vi "Pad Advanced Settings.vi"(8 "Error In":errorcluster) -> (0 "Error Out":errorcluster, 2 "Ok?":bool, 3 "Path to Calibration File":path)   [LabVIEW 2014]
doc: "This VI provides advanced settings like calibration and choosing buttons for game controllers"
uses:
  Controls/Controllers Clusters/Game Pad Buttons Cluster.ctl
  Controls/Controllers Clusters/Pad Advanced Settings States.ctl
  Controls/Controllers Clusters/Game Pad Calibration Cluster.ctl
  Controls/Configuration Files.ctl
  <vilib>/Utility/xml.llb/Read From XML File(string).vi
  <vilib>/Utility/inputDevices.llb/closeJoystick.vi
  <vilib>/Utility/inputDevices.llb/joystickAcquire.vi
panel:
  in  "Load Button":bool
  out "V Axis":i32(slide) scale=-32768.0..32767.0
  out "U Axis":i32(slide) scale=-32768.0..32767.0
  in  "Calibration Button":bool
  out "Buttons":T1
  out "Z Axis Rotation":i32(slide) scale=-32768.0..32767.0
  out "Y Axis Rotation":i32(slide) scale=-32768.0..32767.0
  out "Y Axis":i32(slide) scale=-32768.0..32767.0
  out "X Axis":i32(slide) scale=-32768.0..32767.0
  out "Z Axis":i32(slide) scale=-32768.0..32767.0
  out "X Axis Rotation":i32(slide) scale=-32768.0..32767.0
  in  "Connect Button":bool
  in  "Cancel Button":bool
  in  "OK Button":bool
  # "Game Controllers Advanced Settings"
  # "OK will be available if Path to Calibration File will be correct"
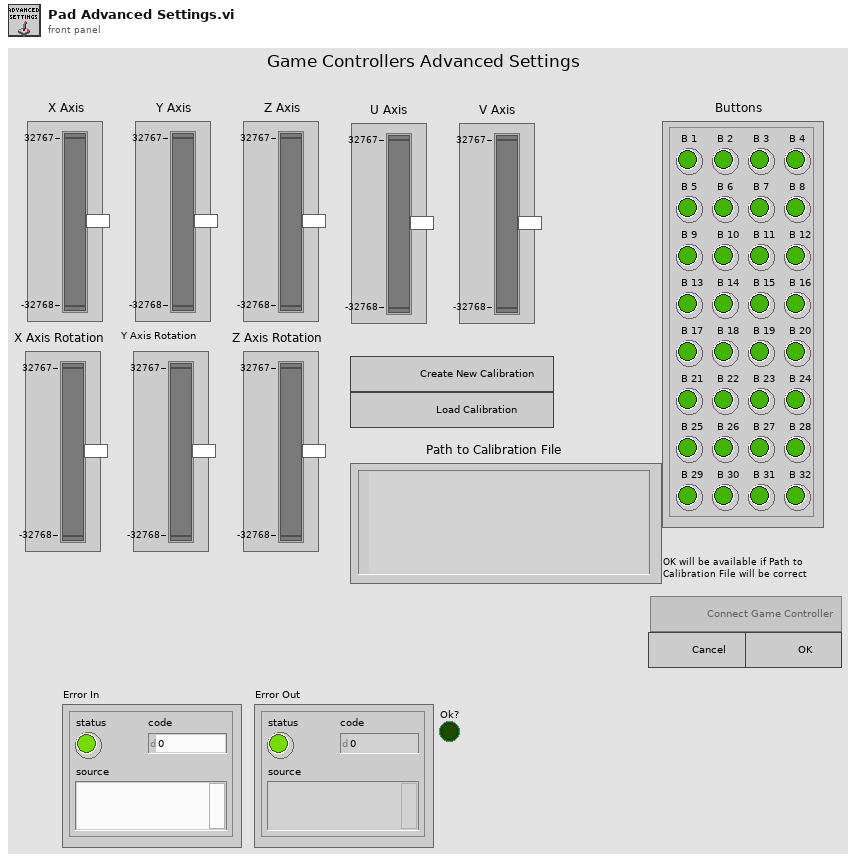
[diagram p1: front panel]
types:
  T1 = typedef "Game Pad Buttons Cluster.ctl" = cluster{"B 1":bool, "B 2":bool, "B 3":bool, "B 4":bool, "B 5":bool, "B 6":bool, "B 7":bool, "B 8":bool, "B 9":bool, "B 10":bool, "B 11":bool, "B 12":bool, "B 13":bool, "B 14":bool, "B 15":bool, "B 16":bool, "B 17":bool, "B 18":bool, "B 19":bool, "B 20":bool, "B 21":bool, "B 22":bool, "B 23":bool, "B 24":bool, "B 25":bool, "B 26":bool, "B 27":bool, "B 28":bool, "B 29":bool, "B 30":bool, "B 31":bool, "B 32":bool}
  T2 = typedef "Pad Advanced Settings States.ctl" = enum16{"Init", "Wait for Event", "Ok", "Cancel"}
  T3 = enum8{"Enabled", "Disabled", "Disabled and Grayed Out"}
  T4 = typedef "Configuration Files.ctl" = string
  T5 = cluster{"X axis":i32, "Y axis":i32, "Z axis":i32, "X axis rotation":i32, "Y axis rotation":i32, "Z axis rotation":i32, "U axis":i32, "V axis":i32}
  T6 = cluster{"button 1":bool, "button 2":bool, "button 3":bool, "button 4":bool, "button 5":bool, "button 6":bool, "button 7":bool, "button 8":bool, "button 9":bool, "button 10":bool, "button 11":bool, "button 12":bool, "button 13":bool, "button 14":bool, "button 15":bool, "button 16":bool, "button 17":bool, "button 18":bool, "button 19":bool, "button 20":bool, "button 21":bool, "button 22":bool, "button 23":bool, "button 24":bool, "button 25":bool, "button 26":bool, "button 27":bool, "button 28":bool, "button 29":bool, "button 30":bool, "button 31":bool, "button 32":bool}
  T7 = typedef "Game Pad Calibration Cluster.ctl" = cluster{"Safety Button Number":u8, "Speed Axis Number":u8, "Speed Axis Max":i32, "Speed Axis Zero":i32, "Back Speed Axis Number":u8, "Back Speed Axis Max":i32, "Back Speed Axis Zero":i32, "Steering Axis Number":u8, "Steering Axis Max":i32, "Steering Axis Zero":i32}
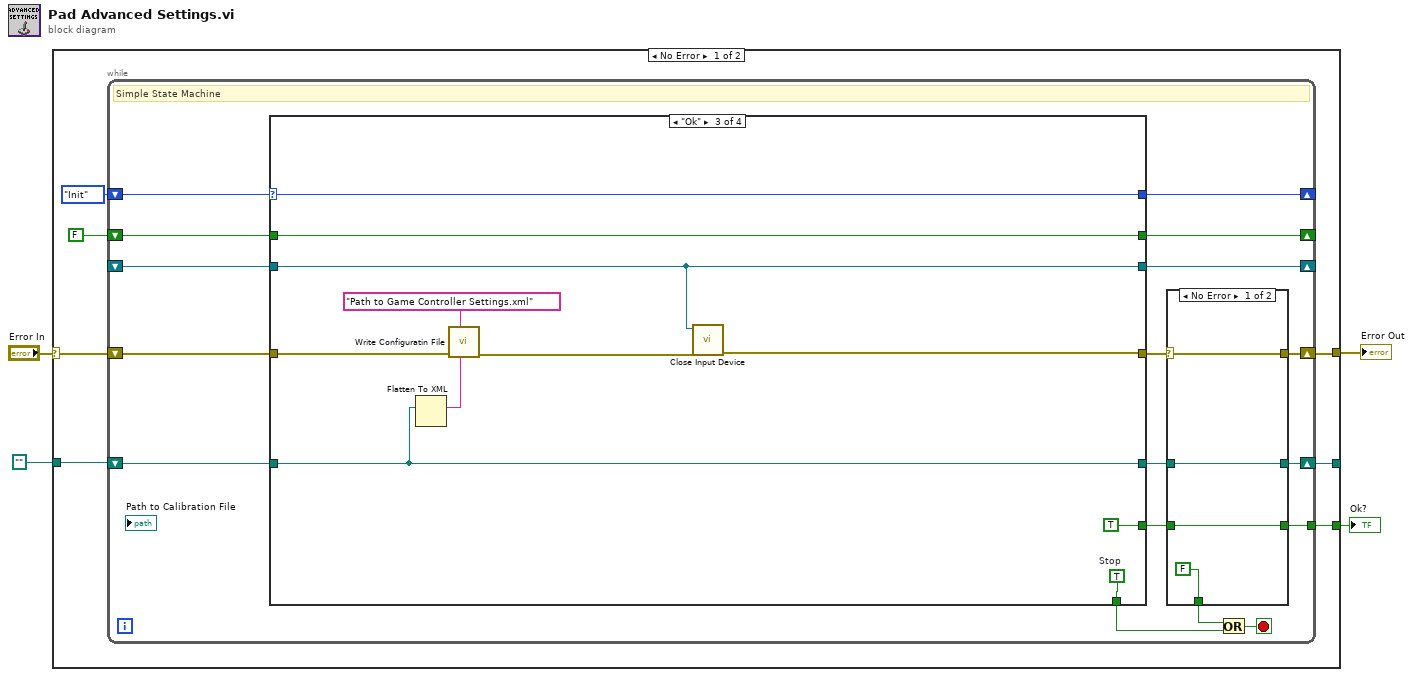
[diagram p0: block diagram]
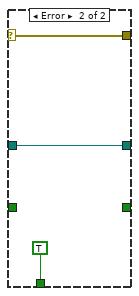
[diagram p2: hidden frame]
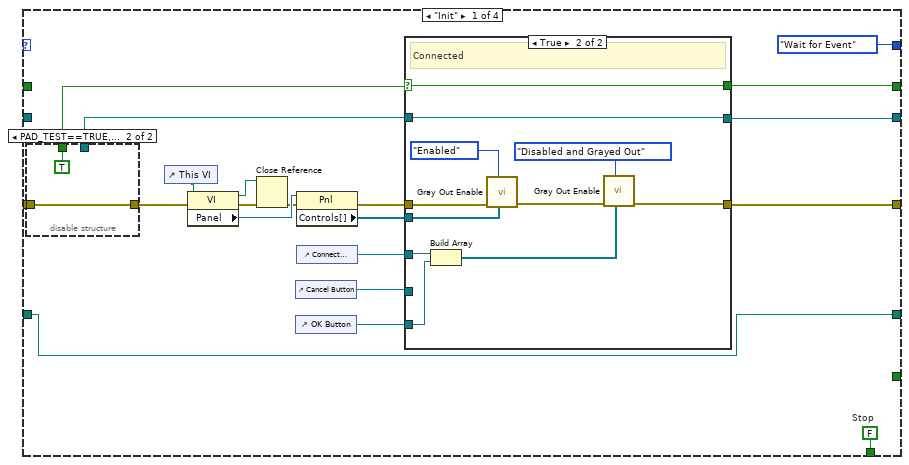
[diagram p3: hidden frame]
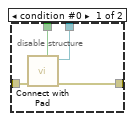
[diagram p4: hidden frame]
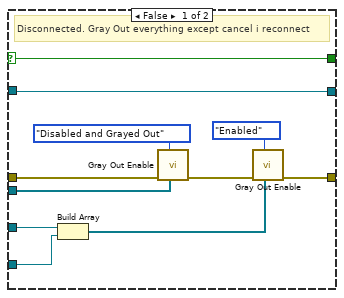
[diagram p5: hidden frame]
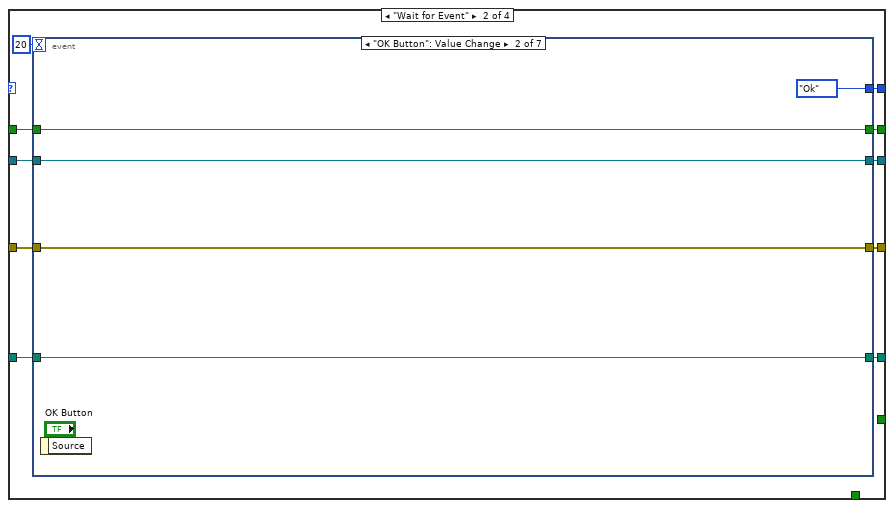
[diagram p6: hidden frame]
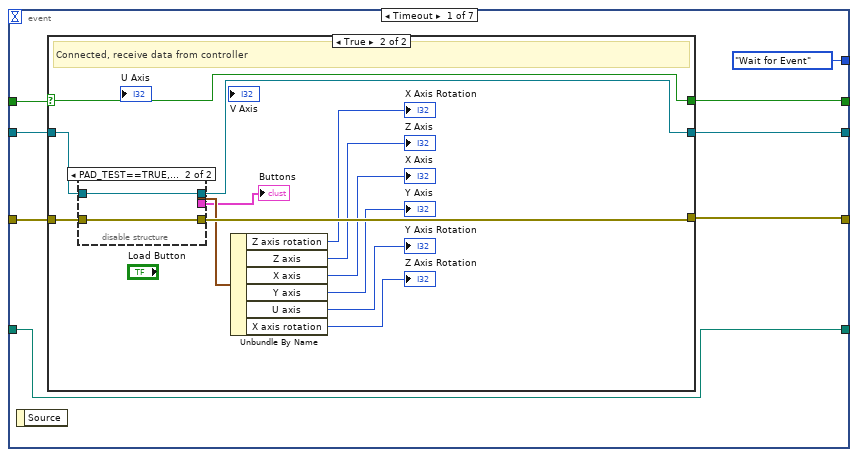
[diagram p7: hidden frame]
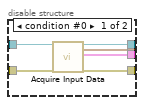
[diagram p9: hidden frame]
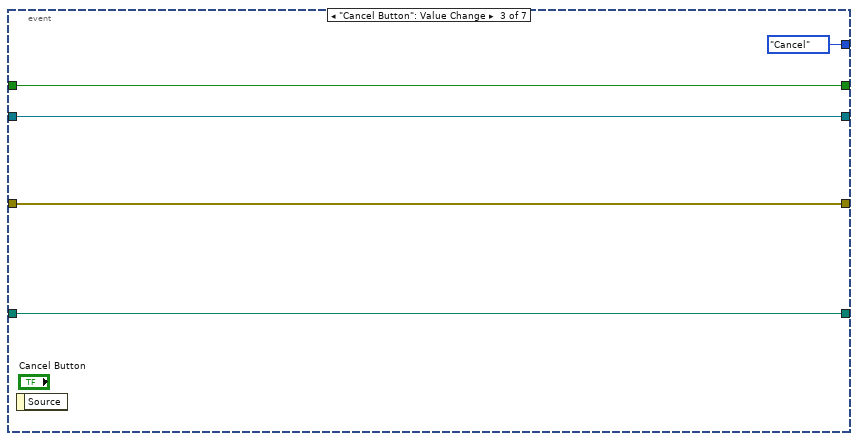
[diagram p10: hidden frame]
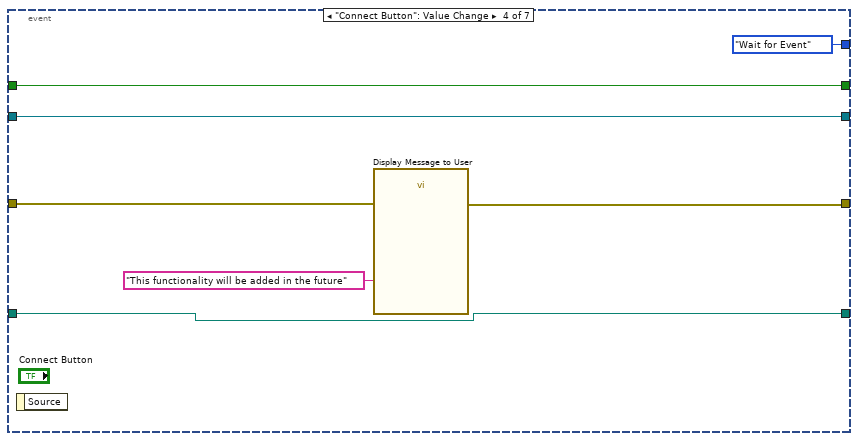
[diagram p11: hidden frame]
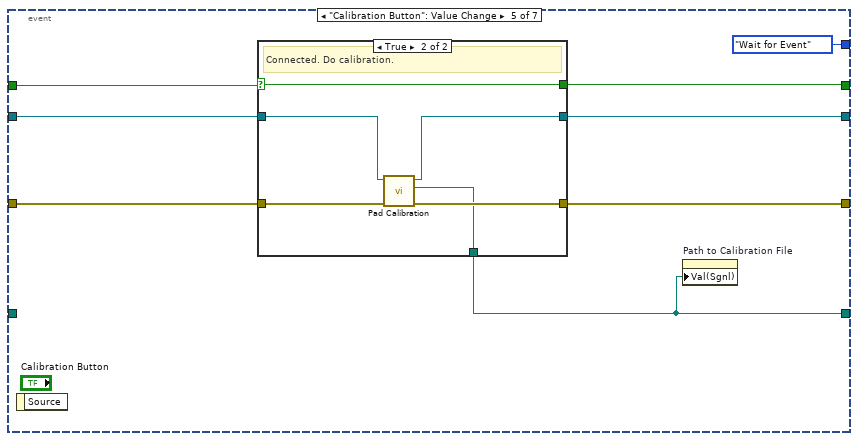
[diagram p12: hidden frame]
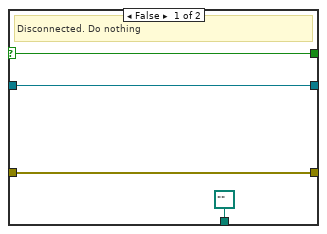
[diagram p13: hidden frame]
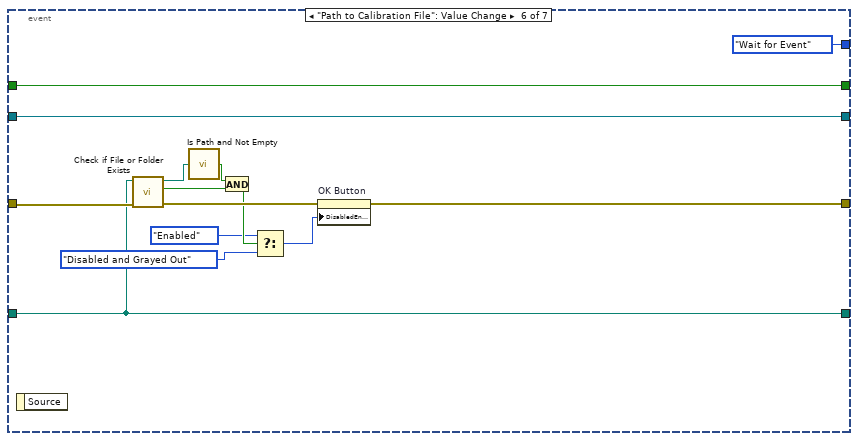
[diagram p14: hidden frame]
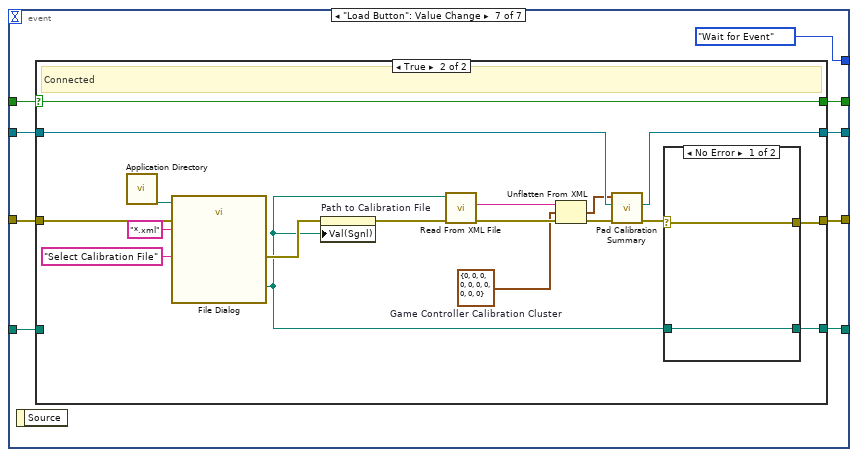
[diagram p15: hidden frame]
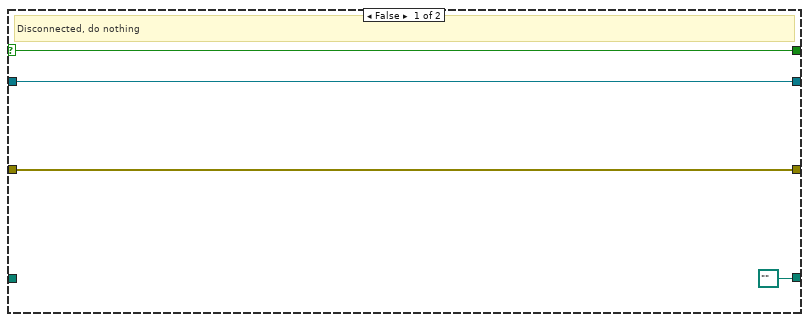
[diagram p16: hidden frame]
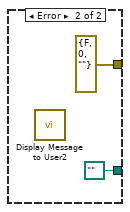
[diagram p17: hidden frame]
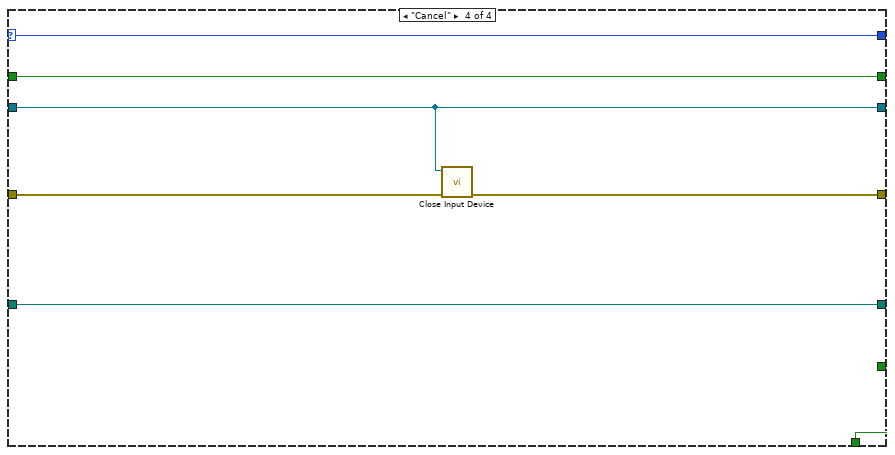
[diagram p18: hidden frame]
diagram:
  n1 = case shown="No Error" "Error In" {
    selector: "Error In" -> [w10 w229]
    tunnel: [w9 w229] -> w3
    tunnel: [w7 w228] -> _
    tunnel: path "" -> [w6 w228]
    tunnel: [w5 _] -> w1
    frame No Error {
      n2 = while {
        shift-right: [w25] -> w9
        shift-left: w10 -> [w14]
        shift-right: [w27] -> _
        shift-left: Pad_Advanced_Settings_States."Init" -> [w28]
        shift-right: [w20] -> _
        shift-left: FALSE -> [w21]
        shift-right: [w18] -> _
        shift-left: _ -> [w19]
        shift-right: [w16] -> w7
        shift-left: w6 -> [w15]
        tunnel: [w12] -> w5
        stop <- w24 stop-if-true
        # "Simple State Machine"
        n3 = case shown="\"Ok\"" w28 {
          selector: w28 -> [_ _ w220 w226]
          tunnel: w14 -> [w53 w93 w215 w223]
          tunnel: [w40 w92 w217 w224] -> w26
          tunnel: [w55 _ w219 w227] -> w22
          tunnel: [Pad_Advanced_Settings_States."Wait for Event" w91 w220 w226] -> w27
          tunnel: w21 -> [_ w90 w218 w225]
          tunnel: [w38 w89 w218 w225] -> w20
          tunnel: [w39 w87 w216 w222] -> w18
          tunnel: w19 -> [_ w88 w216 w222]
          tunnel: [w36 w85 w212 w221] -> w17
          tunnel: w15 -> [w36 w84 w212 w221]
          tunnel: [_ _ TRUE _] -> w13
          frame "Init" {
            w55 = FALSE  # Stop
            n4 = disable-structure shown="PAD_TEST==TRUE, Default" {
              disable-tunnel: w53 -> [w59 w61]
              disable-tunnel: [w58 TRUE ("Connected?")] -> w43
              disable-tunnel: [w57 _] -> w42
              disable-tunnel: [w56 w61] -> w41
              frame condition #0 {
                n5 = call "Connect with Pad.vi"("error in (no error)"=w59) -> ("error out"=w56:errorcluster, "device ID"=w57:refnum<k1>, "Connected?"=w58:bool)  [unwired: 8 in]
              }
              frame condition #1 (active) {
              }
            }
            n6 = control-ref of="This VI"() -> (w48:refnum<vi>)
            n7 = property class="VI"(reference=w48, error in=w41) -> (reference out=w51:refnum<vi>, error out=w50:errorcluster, "Panel"=w52:refnum<vi>)
            n8 = Close Reference(reference=w51, error in (no error)=w50) -> (error out=w49:errorcluster)
            n9 = control-ref of="Cancel Button"() -> (w44:refnum<vi>)
            n10 = control-ref of="OK Button"() -> (w37:refnum<vi>)
            n11 = property class="Pnl"(reference=w52, error in=w49) -> (error out=w47:errorcluster, "Controls[]"=w46:refnum<vi>[])  [unwired: 1 out]
            n12 = control-ref of="Connect Button"() -> (w45:refnum<vi>)
            n13 = case shown="True" w43 {
              selector: w43 -> [w72 w83]
              tunnel: [w72 w83] -> w38
              tunnel: [w71 w82] -> w39
              tunnel: w42 -> [w71 w82]
              tunnel: w47 -> [w65 w81]
              tunnel: [w68 w74] -> w40
              tunnel: w46 -> [w66 w79]
              tunnel: w44 -> [w64 _]
              tunnel: w45 -> [w63 w77]
              tunnel: w37 -> [_ w73]
              frame False {
                # "Disconnected. Gray Out everything except cancel i reconnect"
                n14 = Build Array(w63, w64) -> (w62:refnum<vi>[])
                n15 = call "Gray Out Enable.vi"("Controls[]"=w66, "Disabled"=T3."Disabled and Grayed Out", "Error In"=w65) -> ("Error Out"=w69:errorcluster)  [unwired: 8 in]
                n16 = call "Gray Out Enable.vi"("Controls[]"=w62, "Disabled"=T3."Enabled", "Error In"=w69) -> ("Error Out"=w68:errorcluster)  [unwired: 8 in]
              }
              frame True {
                # "Connected"
                n17 = Build Array(w77, w73) -> (w76:refnum<vi>[])
                n18 = call "Gray Out Enable.vi"("Controls[]"=w79, "Disabled"=T3."Enabled", "Error In"=w81) -> ("Error Out"=w75:errorcluster)  [unwired: 8 in]
                n19 = call "Gray Out Enable.vi"("Controls[]"=w76, "Disabled"=T3."Disabled and Grayed Out", "Error In"=w75) -> ("Error Out"=w74:errorcluster)  [unwired: 8 in]
              }
            }
          }
          frame "Wait for Event" {
            n20 = event shown="[1] \"OK Button\": Value Change" {
              selector: _ -> [_ _ _ _ _ _ _]
              dyn-events: _ -> [_ _ _ _ _ _ _]
              timeout: 20 -> [_ _ _ _ _ _ _]
              tunnel: w93 -> [w96 w130 w134 w142 w145 w174 w182]
              tunnel: [w95 w130 w134 w141 w144 w165 w183] -> w92
              tunnel: [Pad_Advanced_Settings_States."Wait for Event" Pad_Advanced_Settings_States."Ok" Pad_Advanced_Settings_States."Cancel" Pad_Advanced_Settings_States."Wait for Event" Pad_Advanced_Settings_States."Wait for Event" Pad_Advanced_Settings_States."Wait for Event" Pad_Advanced_Settings_States."Wait for Event"] -> w91
              tunnel: [w99 w128 w133 w140 w147 w162 w178] -> w89
              tunnel: w90 -> [w101 w128 w133 w140 w149 w162 w179]
              tunnel: w88 -> [w98 w127 w132 w139 w148 w163 w181]
              tunnel: [w97 w127 w132 w139 w146 w163 w180] -> w87
              tunnel: [w94 w126 w131 w136 w143 w164 w176] -> w85
              tunnel: w84 -> [w94 w126 w131 w136 _ w164 w175]
              event Timeout {
                n21 = event-data() -> ()  [unwired: 1 in, 1 out]
                n22 = case shown="True" w101 {
                  selector: w101 -> [w104 w111]
                  tunnel: [w104 w111] -> w99
                  tunnel: w98 -> [w103 w115]
                  tunnel: [w103 w110] -> w97
                  tunnel: [w102 w116] -> w95
                  tunnel: w96 -> [w102 w117]
                  frame False {
                    # "Not connected, do nothing"
                  }
                  frame True {
                    # "Connected, receive data from controller"
                    n23 = disable-structure shown="PAD_TEST==TRUE, Default" {
                      disable-tunnel: w117 -> [w123 w124]
                      disable-tunnel: [w122 w124] -> w116
                      disable-tunnel: w115 -> [w121 w125]
                      disable-tunnel: [w120 _] -> w114
                      disable-tunnel: [w119 w125] -> w110
                      disable-tunnel: [w118 _] -> w105
                      frame condition #0 {
                        n24 = call-poly <vilib>:"Acquire Input Data.vi"("device ID"=w121, "error in (no error)"=w123) -> ("device ID"=w119:refnum<k1>, "axis info"=w120:T5, "button info"=w118:T6, "error out"=w122:errorcluster)  [unwired: 13 in, 1 out]
                      }
                      frame condition #1 (active) {
                      }
                    }
                    "Buttons" <- w105
                    n25 = Unbundle By Name(w114) -> ("Z axis rotation"=→"X Axis Rotation":i32, "Z axis"=→"Z Axis":i32, "X axis"=→"X Axis":i32, "Y axis"=→"Y Axis":i32, "U axis"=→"Y Axis Rotation":i32, "X axis rotation"=→"Z Axis Rotation":i32)
                  }
                }
              }
              event "OK Button": Value Change {
                n26 = event-data() -> ()  [unwired: 1 in, 1 out]
              }
              event "Cancel Button": Value Change {
                n27 = event-data() -> ()  [unwired: 1 in, 1 out]
              }
              event "Connect Button": Value Change {
                n28 = event-data() -> ()  [unwired: 1 in, 1 out]
                n29 = call "Display Message to User"("error in (no error)"=w142, "Message"="This functionality will be added in the future") -> ("error out"=w141:errorcluster)  [unwired: 8 in, 1 out]
              }
              event "Calibration Button": Value Change {
                n30 = event-data() -> ()  [unwired: 1 in, 1 out]
                n31 = case shown="True" w149 {
                  selector: w149 -> [w154 w160]
                  tunnel: w148 -> [w153 w156]
                  tunnel: [w154 w160] -> w147
                  tunnel: [w153 w157] -> w146
                  tunnel: w145 -> [w152 w159]
                  tunnel: [w152 w158] -> w144
                  tunnel: [path "" ("Path to config file") w155] -> w143
                  frame False {
                    # "Disconnected. Do nothing"
                  }
                  frame True {
                    # "Connected. Do calibration."
                    n32 = call "Pad Calibration.vi"("Error In"=w159, "device ID"=w156) -> ("Error Out"=w158:errorcluster, "Path to config file"=w155:path, "device ID"=w157:refnum<k1>)  [unwired: 7 in]
                  }
                }
                n33 = property on="Path to Calibration File" class="Path"("Val(Sgnl)"=w143) -> ()  [unwired: 2 in, 2 out]
              }
              event "Path to Calibration File": Value Change {
                n34 = event-data() -> ()  [unwired: 1 in, 1 out]
                n35 = call <vilib>:"Check if File or Folder Exists.vi"("error in (no error)"=w174, "path"=w164) -> ("error out"=w170:errorcluster, "file or folder exists?"=w171:bool, "dup path"=w173:path)  [unwired: 7 in]
                n36 = call <vilib>:"Is Path and Not Empty.vi"("path"=w173) -> ("Is Path and Not Empty?"=w172:bool)  [unwired: 4 in]
                n37 = And(x=w172, y=w171) -> (x .and. y?=w169:bool)
                n38 = Select(t=T3."Enabled" ("Disabled"), s=w169, f=T3."Disabled and Grayed Out" ("Disabled")) -> (s? t:f=w166:T3)
                n39 = property on="OK Button" class="Bool"(error in=w170, "DisabledEnum"=w166) -> (error out=w165:errorcluster)  [unwired: 1 in, 1 out]
              }
              event "Load Button": Value Change {
                n40 = event-data() -> ()  [unwired: 1 in, 1 out]
                n41 = case shown="True" w179 {
                  selector: w179 -> [w186 w203]
                  tunnel: [w185 w190] -> w183
                  tunnel: w182 -> [w185 w202]
                  tunnel: w181 -> [w187 w205]
                  tunnel: [w187 w204] -> w180
                  tunnel: [w186 w203] -> w178
                  tunnel: [path "" ("selected path") w188] -> w176
                  tunnel: w175 -> [_ _]
                  frame False {
                    # "Disconnected, do nothing"
                  }
                  frame True {
                    w198 = T7 {"Safety Button Number"=0, "Speed Axis Number"=0, "Speed Axis Max"=0, "Speed Axis Zero"=0, "Back Speed Axis Number"=0, "Back Speed Axis Max"=0, "Back Speed Axis Zero"=0, "Steering Axis Number"=0, "Steering Axis Max"=0, "Steering Axis Zero"=0}  # Game Controller Calibration Cluster
                    # "Connected"
                    n42 = call <vilib>:"Application Directory.vi"() -> ("Application Directory"=w196:path)
                    n43 = call "File Dialog"("start path"=w196, "prompt"="Select Calibration File", "error in"=w202, "pattern (all files)"="*.xml") -> ("selected path"=w189:path, "error out"=w192:errorcluster)  [unwired: 8 in, 2 out]
                    n44 = property on="Path to Calibration File" class="Path"(error in=w192, "Val(Sgnl)"=w189) -> (error out=w193:errorcluster)  [unwired: 1 in, 1 out]
                    n45 = call-poly <vilib>:"Read From XML File.vi"("error in (no error)"=w193, "XML File Path"=w189) -> ("error out"=w201:errorcluster, "XML Elements"=w199:string)  [unwired: 7 in, 1 out]
                    n46 = Unflatten From XML(xml string=w199, type=w198, error in (no error)=w201) -> (value=w197:T7, error out=w200:errorcluster)
                    n47 = call "Pad Calibration Summary.vi"("Error In"=w200, "device ID"=w205, "Calibration Cluster"=w197) -> ("Error Out"=w191:errorcluster, "device ID out"=w204:refnum<k1>)  [unwired: 7 in]
                    n48 = case shown="No Error" w191 {
                      selector: w191 -> [w207 _]
                      tunnel: [w207 errorcluster {"status"=FALSE, "code"=0, "source"=""} ("error constant")] -> w190
                      tunnel: w189 -> [w206 _]
                      tunnel: [w206 path "" ("selected path")] -> w188
                      frame No Error {
                      }
                      frame Error {
                        n49 = call "Display Message to User2"() -> ()  [unwired: 10 in, 2 out]
                      }
                    }
                  }
                }
              }
            }
          }
          frame "Ok" {
            w219 = TRUE  # Stop
            n50 = Flatten To XML(anything=w212) -> (xml string=w211:string)
            n51 = call "Write Configuratin File.vi"("XML String"=w211, "Settings"=T4 "Path to Game Controller Settings.xml", "error in (no error)"=w215) -> ("error out"=w214:errorcluster)  [unwired: 8 in]
            n52 = call-poly <vilib>:"Close Input Device.vi"("error in (no error)"=w214, "device ID"=w216) -> ("error out"=w217:errorcluster)  [unwired: 8 in]
          }
          frame "Cancel" {
            w227 = TRUE  # Stop
            n53 = call-poly <vilib>:"Close Input Device.vi"("error in (no error)"=w223, "device ID"=w222) -> ("error out"=w224:errorcluster)  [unwired: 8 in]
          }
        }
        n54 = case shown="No Error" w26 {
          selector: w26 -> [w32 w35]
          tunnel: [w32 w35] -> w25
          tunnel: [FALSE TRUE] -> w23
          tunnel: w17 -> [w30 w33]
          tunnel: [w30 w33] -> w16
          tunnel: [w29 _] -> w12
          tunnel: w13 -> [w29 _]
          frame No Error {
          }
          frame Error {
          }
        }
        n55 = Or(x=w23, y=w22) -> (x .or. y?=w24:bool)
      }
    }
    frame Error {
    }
  }
  "Error Out" <- w3
  "Ok?" <- w1
